vi "sub_cDAQ_fgv.vi"(7 "cmd":T1, 8 "error in":errorcluster) -> (0 "error out":errorcluster, 3 "data":waveform(dbl)[](array[waveform]) caption="데이터")   [LabVIEW 2016]
uses:
  ctl/strain_ctl.ctl
  <vilib>/DAQmx/read.llb/DAQmx Read (Analog 1D Wfm NChan NSamp).vi
  Global.vi
  <vilib>/DAQmx/miscellaneous.llb/DAQmx Fill In Error Info.vi
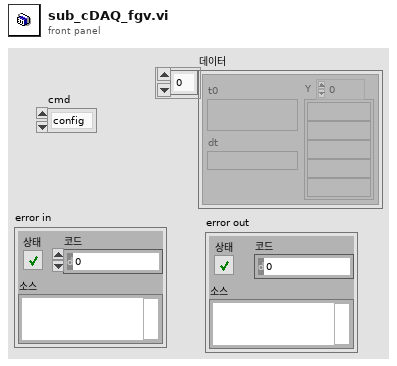
[diagram p1: front panel]
types:
  T1 = typedef "strain_ctl.ctl" = enum16{"config", "start", "read", "close"}
  T2 = cluster{"sampling rate":dbl, "sample to read":dbl}
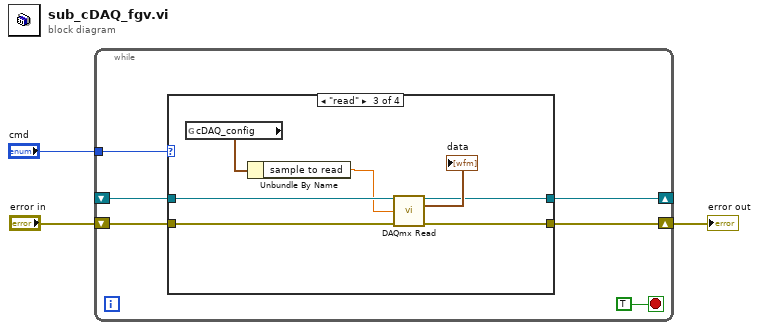
[diagram p0: block diagram]
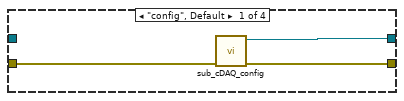
[diagram p2: hidden frame]
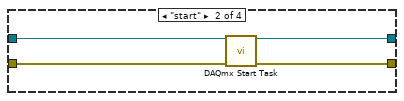
[diagram p3: hidden frame]
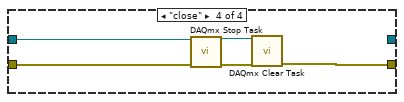
[diagram p4: hidden frame]
diagram:
  n1 = while {
    tunnel: "cmd" -> [w9]
    shift-right: [w7] -> w1
    shift-left: "error in" -> [w8]
    shift-right: [w6] -> _
    shift-left: _ -> [w5]
    stop <- TRUE stop-if-true
    n2 = case shown="\"read\"" w9 {
      tunnel: w8 -> [w12 w16 w21 w26]
      tunnel: [w11 w13 w20 w25] -> w7
      tunnel: [w10 w14 w19 _] -> w6
      tunnel: w5 -> [_ w15 w22 w24]
      frame "config", Default {
        n3 = call "sub_cDAQ_config.vi"("error in"=w12) -> ("error out"=w11:errorcluster, "task out"=w10:refnum<k21>)  [unwired: 9 in]
      }
      frame "start" {
        n4 = call <vilib>:"DAQmx Start Task.vi"("task/channels in"=w15, "error in"=w16) -> ("task out"=w14:refnum<k21>, "error out"=w13:errorcluster)  [unwired: 12 in]
      }
      frame "read" {
        n5 = global read "Global.vi" "cDAQ_config"() -> (w18:T2)
        n6 = Unbundle By Name(w18) -> ("sample to read"=w17:dbl)
        n7 = call-poly <vilib>:"DAQmx Read.vi"("task/channels in"=w22, "number of samples per channel"=w17, "error in"=w21) -> ("task out"=w19:refnum<k21>, "data"=→"data":waveform(dbl)[], "error out"=w20:errorcluster)  [unwired: 10 in]
      }
      frame "close" {
        n8 = call <vilib>:"DAQmx Stop Task.vi"("task/channels in"=w24, "error in"=w26) -> ("task out"=w28:refnum<k21>, "error out"=w27:errorcluster)  [unwired: 12 in]
        n9 = call <vilib>:"DAQmx Clear Task.vi"("task in"=w28, "error in"=w27) -> ("error out"=w25:errorcluster)  [unwired: 13 in]
      }
    }
  }
  "error out" <- w1
